vi "Gaussian Peak Fit.vi"(0 "Y":dbl[](array[numeric]), 1 "initial guess":T2={"initial amplitude"=nan, "initial center"=nan, "initial standard deviation"=nan, "offset"=nan}, 5 "X":dbl[](array[numeric]), 7 "Weight":dbl[](array[numeric]), 9 "tolerance":dbl=0.0001 format="%#_3g", 11 "method":T3 items=["Least Square", "Least Absolute Residual", "Bisquare"], 12 "parameter bounds":T1={"amp min"=-inf, "amp max"=inf, "center min"=-inf, "center max"=inf, "deviation min"=-inf, "deviation max"=inf, "offset min"=0.0, "offset max"=0.0}) -> (3 "offset":dbl, 4 "Best Gaussian Fit":dbl[](array[numeric]), 6 "amplitude":dbl, 8 "center":dbl, 10 "standard deviation":dbl, 14 "residue":dbl, 15 "error":i32)   [LabVIEW 2014, in "NI_AALPro.lvlib"]
doc: "Returns the Gaussian fit of a data set (<B>X</B>, <B>Y</B>) using the Least Square, Least Absolute Residual, or Bisquare method."
uses:
  NI_AALPro.lvlib
  Curve Fitting Criteria.ctl
  lvanlys.dll
panel:
  # "Constrained Gaussian Peak Fit"
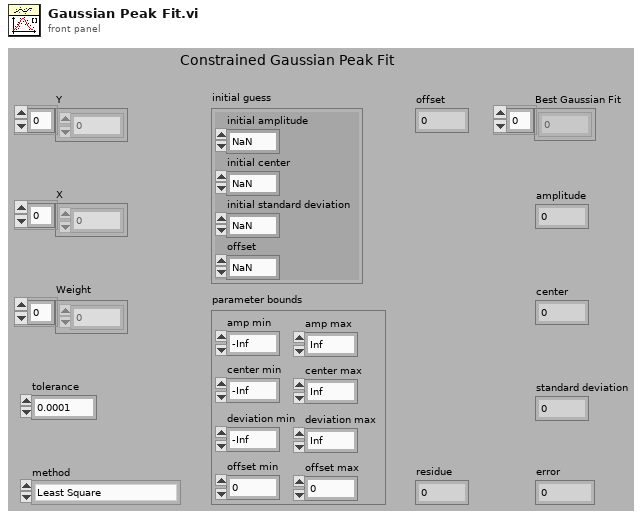
[diagram p1: front panel]
types:
  T1 = cluster{"amp min":dbl, "amp max":dbl, "center min":dbl, "center max":dbl, "deviation min":dbl, "deviation max":dbl, "offset min":dbl, "offset max":dbl}
  T2 = cluster{"initial amplitude":dbl, "initial center":dbl, "initial standard deviation":dbl, "offset":dbl}
  T3 = typedef "NI_AALPro.lvlib/Curve Fitting Criteria.ctl" = u16
  T4 = cluster{"initial amplitude":dbl, "initial center":dbl, "initial standard deviation":dbl}
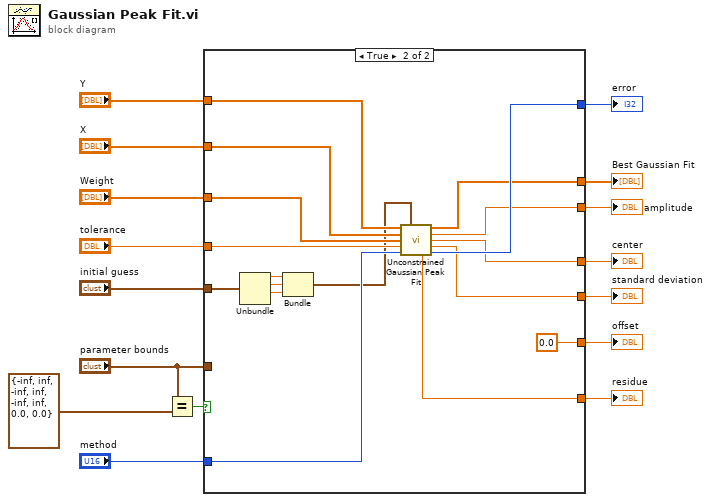
[diagram p0: block diagram]
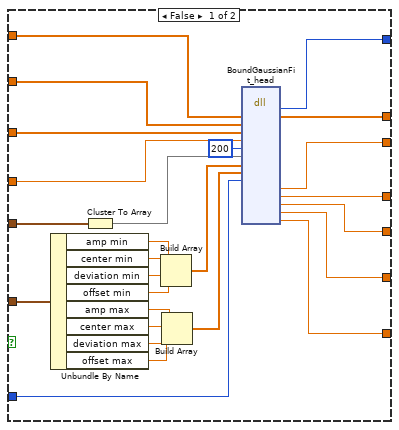
[diagram p2: hidden frame]
diagram:
  n1 = Equal?(x="parameter bounds", y=T1 {"amp min"=-inf, "amp max"=inf, "center min"=-inf, "center max"=inf, "deviation min"=-inf, "deviation max"=inf, "offset min"=0.0, "offset max"=0.0} ("parameter bounds 2")) -> (x = y?=w1:bool)
  n2 = case shown="True" w1 {
    tunnel: "initial guess" -> [w42 w47]
    tunnel: "X" -> [w41 w58]
    tunnel: "Weight" -> [w40 w57]
    tunnel: "tolerance" -> [w39 w56]
    tunnel: "method" -> [w36 w55]
    tunnel: [w35 w53] -> w11
    tunnel: [w34 w52] -> w10
    tunnel: [w33 w51] -> w9
    tunnel: [w32 w50] -> w8
    tunnel: [w31 0.0 ("offset")] -> w7
    tunnel: [w30 w48] -> w6
    tunnel: "parameter bounds" -> [w29 _]
    tunnel: "Y" -> [w18 w59]
    tunnel: [w17 w54] -> w4
    frame False {
      n3 = Unbundle By Name(w29) -> ("amp min"=w28:dbl, "center min"=w27:dbl, "deviation min"=w26:dbl, "offset min"=w25:dbl, "amp max"=w24:dbl, "center max"=w23:dbl, "deviation max"=w22:dbl, "offset max"=w21:dbl)
      n4 = Cluster To Array(cluster=w42) -> (array=w37:dbl[])
      n5 = Build Array(w28, w27, w26, w25) -> (w20:dbl[])
      n6 = Build Array(w24, w23, w22, w21) -> (w19:dbl[])
      n7 = dll-call lib="C:/Program Files (x86)/National Instruments/LabVIEW 2014/resource/lvanlys.*" fn="BoundGaussianFit_head"("y"=w18, "x"=w41, "weight"=w40, "tolerance"=w39, "maxIter"=200, "intial coef"=w37, "minBound"=w20, "maxBound"=w19, "algorithm"=w36) -> ("return type"=w17:i32, "y"=w35:dbl[], "amp"=w34:dbl, "center"=w33:dbl, "deviation"=w32:dbl, "offset"=w31:dbl, "mse"=w30:dbl)  [unwired: 9 in, 9 out]
    }
    frame True {
      n8 = Unbundle(w47) -> ("initial amplitude"=w46:dbl, "initial center"=w44:dbl, "initial standard deviation"=w43:dbl)  [unwired: 1 out]
      n9 = Bundle("initial amplitude"=w46, "initial center"=w44, "initial standard deviation"=w43) -> (w45:T4)  [unwired: 1 out]
      n10 = call "Unconstrained Gaussian Peak Fit.vi"("Y"=w59, "initial guess"=w45, "X"=w58, "Weight"=w57, "tolerance"=w56, "method"=w55) -> ("Best Gaussian Fit"=w53:dbl[], "amplitude"=w52:dbl, "center"=w51:dbl, "standard deviation"=w50:dbl, "residue"=w48:dbl, "error"=w54:i32)  [unwired: 4 out]
    }
  }
  "center" <- w9
  "amplitude" <- w10
  "Best Gaussian Fit" <- w11
  "standard deviation" <- w8
  "error" <- w4
  "residue" <- w6
  "offset" <- w7
